vi "Serial Write.vi"() -> ()   [LabVIEW 2023]
doc: "This example opens two VISA resources and configures one COM port to perform a write operation and the other COM port to perform a read operation. This VI will wait until the specified number of bytes is received at the port or until a termination character is read.\n\nThis example allows you perform diagnostic tests on your ports. You can use this example to perform a wrap-back test. Both serial ports must have the same basic configuration parameters. You can connect two of the ports using a null modem cable, which effectively connects one port's RX lines to the other port's TX lines. If you use a straight-through cable, one port's RX lines will be connected to the other port's RX lines, and you cannot communicate between the two ports."
uses:
  C:/Program Files (x86)/National Instruments/LabVIEW 2023/examples/Instrument IO/Serial/support/Serial - Settings.ctl
  <vilib>/Instr/_visa.llb/VISA Configure Serial Port (Instr).vi
panel:
  in  "stop":bool
  out "read buffer":string
  out "Frecuency 2":string
  out "Frecuncy 1":string
  in  "Frecuency 2":dbl(slide) scale=0.0..3000.0
  in  "Frecuency 1":dbl(slide) scale=0.0..3000.0
  in  "Termination Character":u8=10 format="%.0x"
  in  "End Write on Termination Character?":bool=TRUE
  in  "Serial Settings (write)":T1={"baud rate"=9600, "data bits"=8, "parity"=enum."None", "stop bits"=10, "flow control"=0} {"flow control" items=["None"=0, "XON/XOFF"=1, "RTS/CTS"=2, "DTR/DSR"=4]; "stop bits" items=["1.0"=10, "1.5"=15, "2.0"=20]; "data bits" min=5 max=8 step=1; "baud rate" items=["75"=75, "110"=110, "134"=134, "150"=150, "300"=300, "600"=600, "1200"=1200, "1800"=1800, "2400"=2400, "4800"=4800, "7200"=7200, "9600"=9600, "14400"=14400, "19200"=19200, "28800"=28800, "38400"=38400, "56000"=56000, "57600"=57600, "115200"=115200, "128000"=128000, "230400"=230400]}
  out "bytes written":u32
  in  "VISA Resource (write)":refnum<visa-resource-name>="COM1"
  # "Overview: Demonstrates the use of the VISA functions to communicate between two different serial devices.\nRequirements: NI-VISA Driver, two serial devices\nInstructions:\n1. Ensure the resources specified by VISA Resource (write) and VISA Resource (read) are valid serial devices.\n2. Connect a null modem RS-232 or RS-485/422 cable between the 2 ports.\n3. Run the VI.\n4. If your two devices are connected properly, you should see the Read String value match the Write String value."
  # "0xA is equivalent to a '\\n' character, which is a line feed.\nAnd 44--> 0X2C is equivalent to ','."
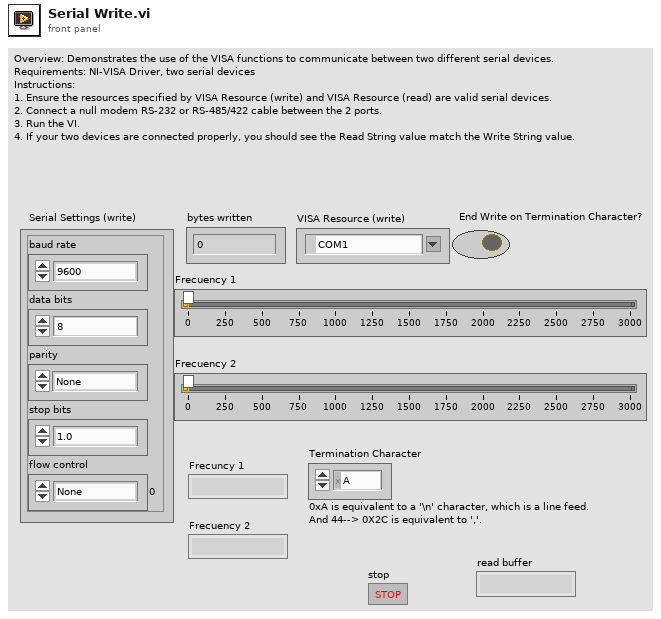
[diagram p1: front panel]
types:
  T1 = typedef "Serial - Settings.ctl" = cluster{"baud rate":u32, "data bits":u16, "parity":enum16{"None", "Odd", "Even", "Mark", "Space"}, "stop bits":u16, "flow control":u16}
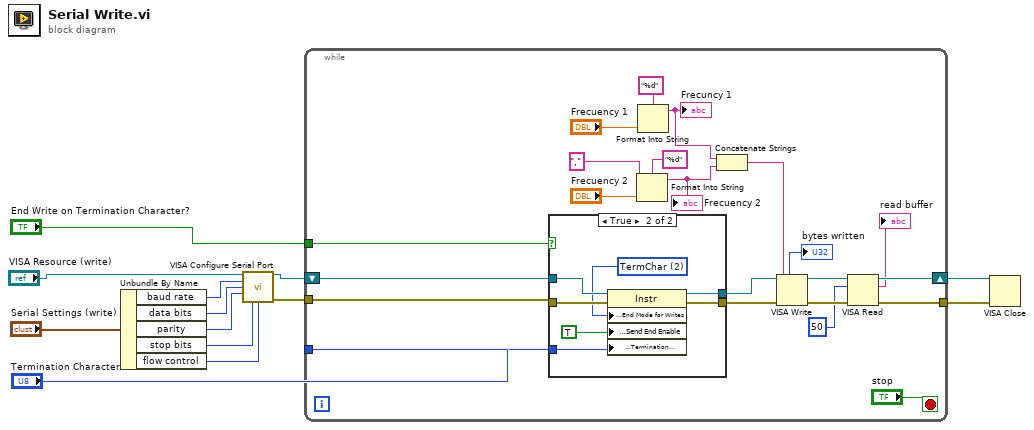
[diagram p0: block diagram]
diagram:
  n1 = Unbundle By Name("Serial Settings (write)") -> ("baud rate"=w8:u32, "data bits"=w7:u16, "parity"=w6:enum16{"None", "Odd", "Even", "Mark", "Space"}, "stop bits"=w5:u16, "flow control"=w4:u16)
  n2 = call-poly "VISA Configure Serial Port"("VISA resource name"="VISA Resource (write)", "baud rate (9600)"=w8, "data bits (8)"=w7, "parity (0:none)"=w6, "stop bits (10: 1 bit)"=w5, "flow control (0:none)"=w4) -> ("VISA resource name out"=w2:refnum<visa-resource-name>, "error out"=w3:errorcluster)  [unwired: 3 in, 5 out]
  n3 = while {
    tunnel: "End Write on Termination Character?" -> [w32]
    tunnel: "Termination Character" -> [w31]
    shift-right: [w21] -> w10
    shift-left: w2 -> [w35]
    tunnel: w3 -> [w15]
    tunnel: [w14] -> w1
    stop <- "stop" stop-if-true
    n4 = case shown="True" w32 {
      tunnel: w35 -> [w36 w44]
      tunnel: w15 -> [w37 w43]
      tunnel: [w36 w42] -> w34
      tunnel: [w37 w41] -> w33
      tunnel: w31 -> [_ w39]
      frame False {
      }
      frame True {
        w40 = u16 2 items=["None", "LastBit", "TermChar", "Break"] ("Serial Settings:Serial End Mode for Writes")
        n5 = property class="Instr"(reference=w44, error in=w43, "Serial Settings:End Mode for Writes"=w40, "Message Based Settings:Send End Enable"=TRUE, "Message Based Settings:Termination Character"=w39) -> (reference out=w42:refnum<visa-resource-name>, error out=w41:errorcluster)
      }
    }
    n6 = Format Into String(format string="%d", initial string=",", "Frecuency 2") -> (resulting string=w23:string)  [unwired: 1 in, 1 out]
    "Frecuency 2" <- w23
    n7 = Format Into String(format string="%d", "Frecuency 1") -> (resulting string=w24:string)  [unwired: 2 in, 1 out]
    "Frecuncy 1" <- w24
    n8 = Concatenate Strings(w24, w23) -> (w30:string)
    n9 = VISA Write(VISA resource name=w34, write buffer=w30, error in (no error)=w33) -> (VISA resource name out=w22:refnum<visa-resource-name>, return count=→"bytes written":u32, error out=w20:errorcluster)
    n10 = VISA Read(VISA resource name=w22, byte count=u32 50, error in (no error)=w20) -> (VISA resource name out=w21:refnum<visa-resource-name>, read buffer=→"read buffer":string, error out=w14:errorcluster)  [unwired: 1 out]
  }
  n11 = VISA Close(VISA resource name=w10, error in (no error)=w1) -> ()  [unwired: 1 out]
